vi "Error.vi"(10 "Newton (N)":dbl) -> (2 "Error":dbl)   [LabVIEW 2014]
panel:
  out "x*y":dbl
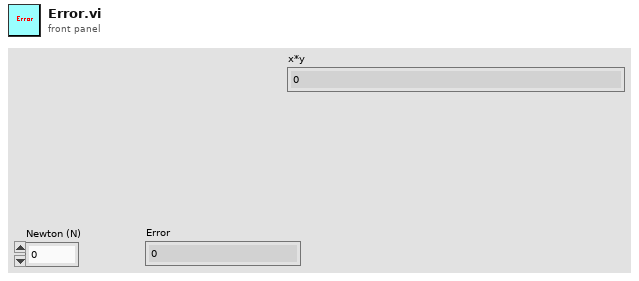
[diagram p1: front panel]
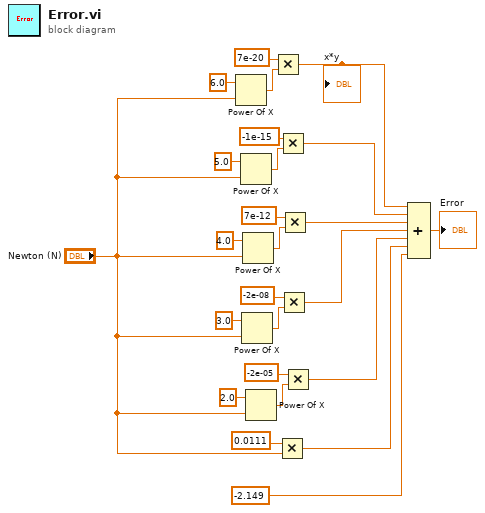
[diagram p0: block diagram]
diagram:
  n1 = Power Of X(1:"Newton (N)", 2:6.0 ("y")) -> (0:w23:dbl)
  n2 = Power Of X(1:"Newton (N)", 2:5.0 ("y")) -> (0:w22:dbl)
  n3 = Power Of X(1:"Newton (N)", 2:3.0 ("y")) -> (0:w16:dbl)
  n4 = Power Of X(1:"Newton (N)", 2:4.0 ("y")) -> (0:w17:dbl)
  n5 = Power Of X(1:"Newton (N)", 2:2.0 ("y")) -> (0:w11:dbl)
  n6 = Multiply(x=7e-20, y=w23) -> (x*y=w2:dbl)
  "x*y" <- w2
  n7 = Multiply(x=0.0111, y="Newton (N)") -> (x*y=w5:dbl)
  n8 = Multiply(x=-1e-15, y=w22) -> (x*y=w9:dbl)
  n9 = Multiply(x=-2e-08, y=w16) -> (x*y=w7:dbl)
  n10 = Multiply(x=7e-12, y=w17) -> (x*y=w8:dbl)
  n11 = Multiply(x=-2e-05, y=w11) -> (x*y=w6:dbl)
  n12 = Compound Arithmetic op=ADD(w2, w9, w8, w7, w6, w5, -2.149) -> (→"Error":dbl)
